vi "Monitor.vi"(8 "Error Out 2":errorcluster, 9 "notifier out 2":refnum<notifier>, 10 "filename":string="Test") -> (0 "Error Out":errorcluster, 2 "output file path":path)   [LabVIEW 2016]
uses:
  <userlib>/Levylab/Lockin-Multichannel/Instrument.Lockin/Instrument.Lockin.lvclass
  <vilib>/Utility/file.llb/Write Delimited Spreadsheet (string).vi
  <userlib>/Levylab/LV to ITX/Main/LV to DAT 1D.vi
  <userlib>/Levylab/LV to ITX/LVtoITX.lvclass
panel:
  out "latest notification":bool
  in  "Lockin IP Address UwU":string="130.49.180.51"
  in  "Tab Control":enum32{"Conductance"}(tab)
  in  "Voltage Pairs (+, -,...)":i32[][](array[numeric])=[[0, 1, 1, 2], [2, 3, 4, 3]]
  in  "Current (I-)":i32
  out "Two Terminal Conductance":cluster{"Y":dbl[], "Y":dbl[]}[](graph) caption="XY Graph"
  out "Four Terminal Resistance":cluster{"Y":dbl[], "Y":dbl[]}[](graph) caption="XY Graph"
  in  "Excitation voltage":dbl=0.1
  in  "Reset":bool
  in  "Diff Voltage?":bool
  out "ALL G2T":dbl[][](graph)
  in  "wait (ms)":u32=60
  out "Humidity":dbl=35.08
  out "Temperature":dbl=27.13
  in  "error in (no error)":errorcluster
  in  "stop":bool
  in  "base path":path=path "C:/Users/ansom/Desktop/Monitor/20180205"
  in  "Comments":string="Test"
  in  "folder name":string="monitor cond"
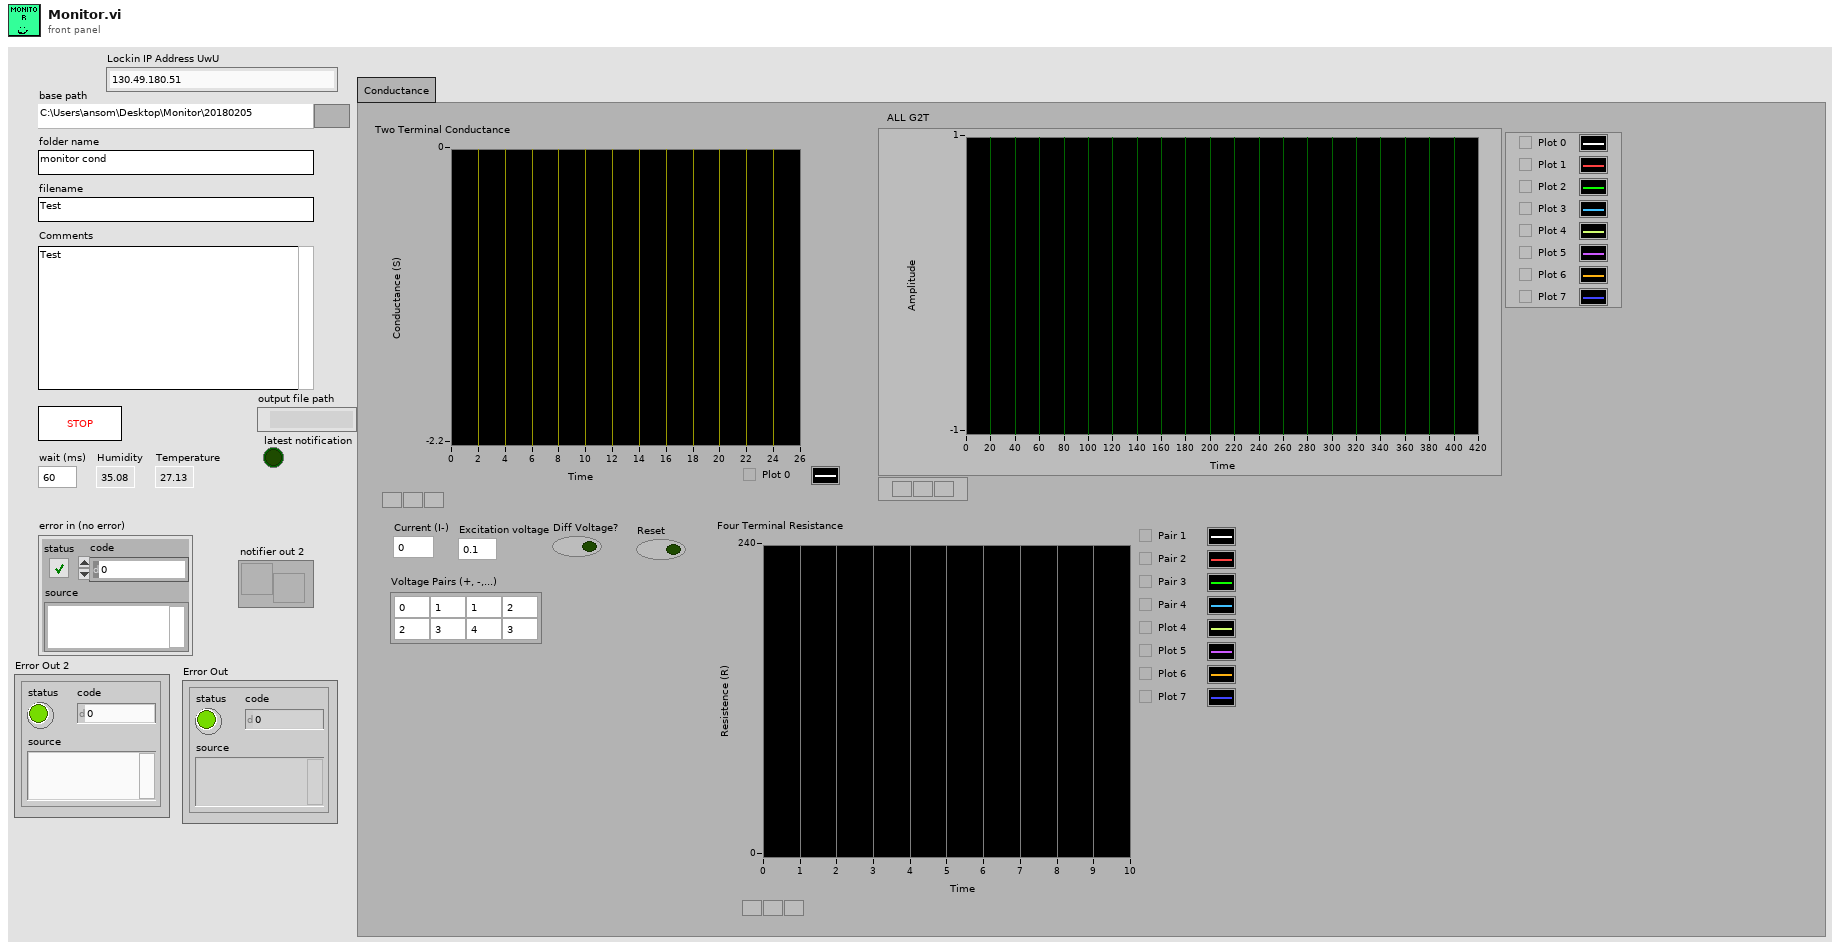
[diagram p1: front panel]
types:
  T1 = enum32{"Bad", "Idle", "Run top level", "Running"}
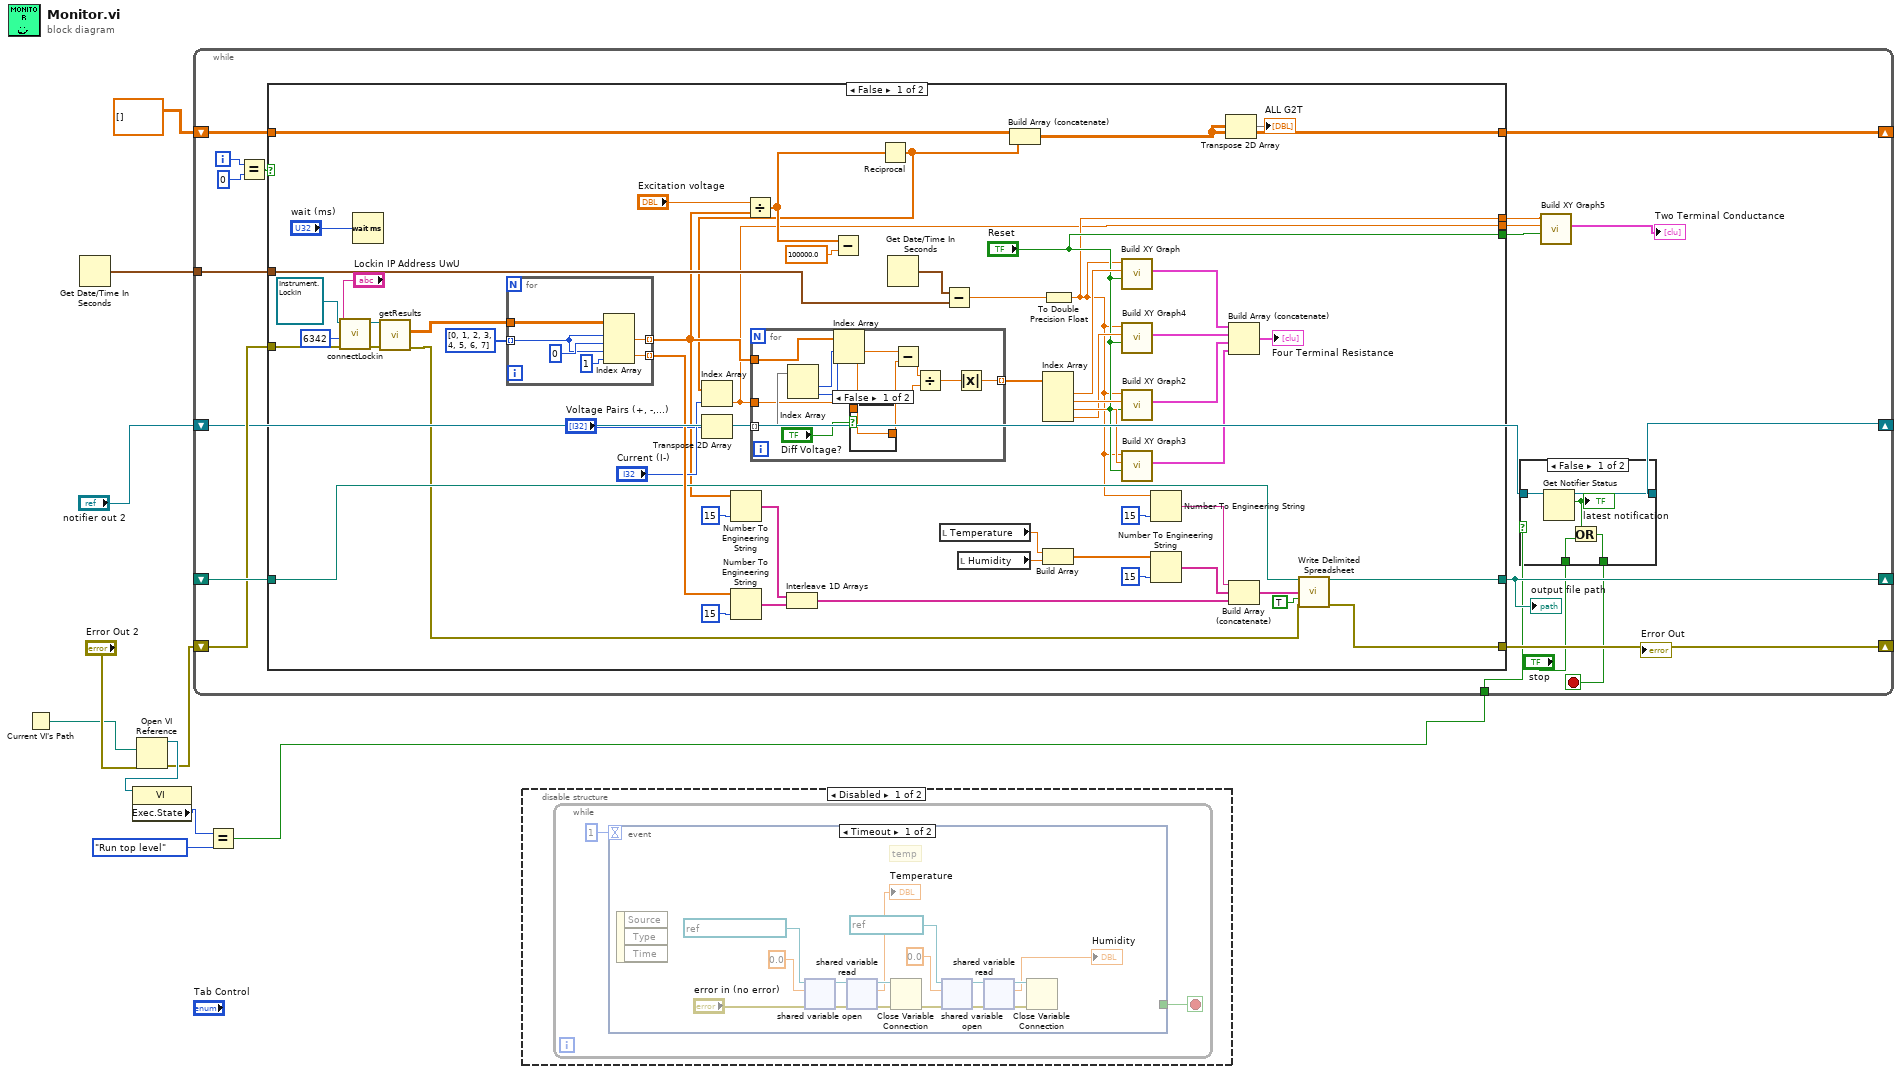
[diagram p0: block diagram]
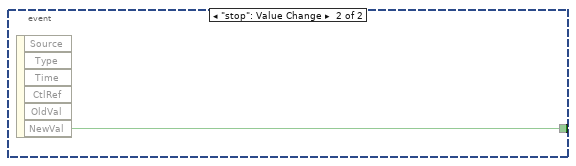
[diagram p2: hidden frame]
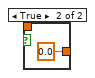
[diagram p5: hidden frame]
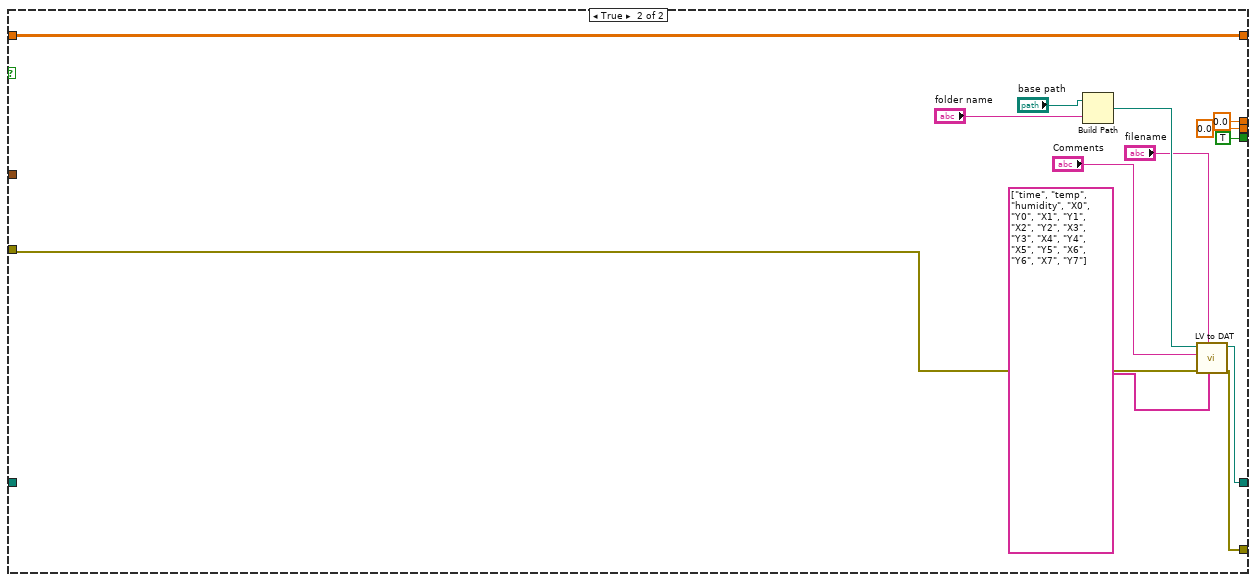
[diagram p6: hidden frame]
diagram:
  n1 = Current VI's Path() -> (path=w1:path)
  n2 = Get Date/Time In Seconds() -> (seconds since 1Jan1904=w11:timestamp)
  n3 = Open VI Reference(vi path=w1, error in (no error)="Error Out 2") -> (vi reference=w7:refnum<vi>, error out=w2:errorcluster)  [unwired: 4 in]
  n4 = property class="VI"(reference=w7) -> ("Exec.State"=w5:T1)  [unwired: 1 in, 2 out]
  n5 = Equal?(x=w5, y=T1."Run top level" ("Execution:State")) -> (x = y?=w3:bool)
  n6 = while {
    shift-right: [w21] -> _
    shift-left: _ -> [w27]
    tunnel: w11 -> [w26]
    shift-right: [w24] -> _
    shift-left: dbl[][] [] ("transposed array") -> [w25]
    shift-right: [w22] -> w9
    shift-left: w2 -> [w23]
    shift-right: [w17] -> _
    shift-left: "notifier out 2" -> [w18]
    tunnel: w3 -> [w19]
    i -> [w30]
    stop <- w16 stop-if-true
    n7 = Equal?(x=w30, y=0) -> (x = y?=w28:bool)
    n8 = case shown="False" w28 {
      tunnel: [w82 w123] -> w21
      tunnel: w27 -> [w85 _]
      tunnel: w26 -> [w58 _]
      tunnel: w25 -> [w50 w118]
      tunnel: [w49 w118] -> w24
      tunnel: w23 -> [w46 w116]
      tunnel: [w45 w117] -> w22
      tunnel: ["Reset" TRUE ("Reset")] -> w15
      tunnel: [w43 0.0] -> w14
      tunnel: [w42 0.0] -> w13
      frame False {
        n9 = call <userlib>:"connectLockin.vi"("error in (no error)"=w46, "Port"=u16 6342, "Address"="Lockin IP Address UwU", "Instrument.Lockin in"=refnum<class "Instrument.Lockin.lvclass"> refnum) -> ("error out"=w39:errorcluster, "Instrument.Lockin out"=w38:refnum<class "Instrument.Lockin.lvclass">)  [unwired: 6 in]
        n10 = Wait (ms)(milliseconds to wait="wait (ms)") -> ()  [unwired: 1 out]
        n11 = call <userlib>:"getResults.vi"("error in (no error)"=w39, "Instrument.Lockin in"=w38) -> ("error out"=w40:errorcluster, "Results"=w41:dbl[][])  [unwired: 6 in, 2 out]
        n12 = for {
          tunnel: w41 -> [w109]
          tunnel: i32[] [0, 1, 2, 3, 4, 5, 6, 7] ("Lockins") -> [w110] mode=indexing
          tunnel: [w107] -> w51 mode=indexing
          tunnel: [w108] -> w86 mode=indexing
          n13 = Index Array(array=w109, index (row) #1=w110, index (col) #1=0 ("disabled index (col)"), index (row) #2=w110, index (col) #2=1 ("disabled index (col)")) -> (element #1=w107:dbl, element #2=w108:dbl)
        }
        n14 = Transpose 2D Array(2D array="Voltage Pairs (+, -,...)") -> (transposed array=w71:i32[][])
        n15 = Number To Engineering String(2:i16 15 ("precision (6)"), 4:w51) -> (0:w89:string[])  [unwired: 2 out]
        n16 = Number To Engineering String(2:i16 15 ("precision (6)"), 4:w86) -> (0:w88:string[])  [unwired: 2 out]
        n17 = Divide(x="Excitation voltage", y=w51) -> (x/y=w55:dbl[])
        n18 = Interleave 1D Arrays(w89, w88) -> (w87:string[])
        n19 = Subtract(x=w55, y=100000.0) -> ()  [unwired: 1 out]
        n20 = Reciprocal(x=w55) -> (1/x=w47:dbl[])
        n21 = Index Array(array=w47, index="Current (I-)") -> (element=w42:dbl)
        n22 = for {
          tunnel: w71 -> [w104] mode=indexing
          tunnel: w51 -> [w103]
          tunnel: w42 -> [w99]
          tunnel: [w96] -> w70 mode=indexing
          n23 = Index Array(array=w104) -> (element #1=w102:i32, element #2=w101:i32)  [unwired: 2 in]
          n24 = Index Array(array=w103, index #1=w102, index #2=w101) -> (element #1=w100:dbl, element #2=w93:dbl)
          n25 = case shown="False" "Diff Voltage?" {
            tunnel: [w105 0.0] -> w94
            tunnel: w93 -> [w105 _]
            frame False {
            }
            frame True {
            }
          }
          n26 = Subtract(x=w100, y=w94) -> (x-y=w98:dbl)
          n27 = Divide(x=w98, y=w99) -> (x/y=w97:dbl)
          n28 = Absolute Value(x=w97) -> (abs(x)=w96:dbl)
        }
        n29 = Get Date/Time In Seconds() -> (seconds since 1Jan1904=w59:timestamp)
        n30 = local read "Temperature"() -> (w81:dbl)
        n31 = Subtract(x=w59, y=w58) -> (x-y=w57:dbl)
        n32 = local read "Humidity"() -> (w80:dbl)
        n33 = Build Array (concatenate)(w50, w47) -> (w49:dbl[][])
        n34 = Index Array(array=w70) -> (element #1=w69:dbl, element #2=w68:dbl, element #3=w67:dbl, element #4=w66:dbl)  [unwired: 4 in]
        n35 = Build Array(w81, w80) -> (w75:dbl[])
        n36 = To Double Precision Float(number=w57) -> (double precision float=w43:dbl)
        n37 = call "Build XY Graph"("Reset"="Reset", "Y Input"=w69, "X Input"=w43) -> ("XY Graph"=w65:cluster{"Y":dbl[], "Y":dbl[]}[])  [unwired: 2 in, 6 out]
        n38 = call "Build XY Graph4"("Reset"="Reset", "Y Input"=w66, "X Input"=w43) -> ("XY Graph"=w64:cluster{"Y":dbl[], "Y":dbl[]}[])  [unwired: 2 in, 6 out]
        n39 = call "Build XY Graph2"("Reset"="Reset", "Y Input"=w68, "X Input"=w43) -> ("XY Graph"=w63:cluster{"Y":dbl[], "Y":dbl[]}[])  [unwired: 2 in, 6 out]
        n40 = call "Build XY Graph3"("Reset"="Reset", "Y Input"=w67, "X Input"=w43) -> ("XY Graph"=w62:cluster{"Y":dbl[], "Y":dbl[]}[])  [unwired: 2 in, 6 out]
        n41 = Number To Engineering String(2:i16 15 ("precision (6)"), 4:w43) -> (0:w77:string)  [unwired: 2 out]
        n42 = Number To Engineering String(2:i16 15 ("precision (6)"), 4:w75) -> (0:w74:string[])  [unwired: 2 out]
        n43 = Transpose 2D Array(2D array=w49) -> (transposed array=→"ALL G2T":dbl[][])
        n44 = Build Array (concatenate)(w65, w64, w63, w62) -> (→"Four Terminal Resistance":cluster{"Y":dbl[], "Y":dbl[]}[])
        n45 = Build Array (concatenate)(w77, w74, w87) -> (w83:string[])
        n46 = call-poly <vilib>:"Write Delimited Spreadsheet.vi"("file path (dialog if empty)"=w85, "1D data"=w83, "append to file? (new file:F)"=TRUE, "error in (no error)"=w40) -> ("new file path (Not A Path if cancelled)"=w82:path, "error out"=w45:errorcluster)  [unwired: 10 in]
      }
      frame True {
        n47 = Build Path(base path="base path", name or relative path="folder name") -> (appended path=w122:path)
        n48 = call-poly <userlib>:"LV to DAT.vi"("wavenames (.Vx, etc)"=string[] ["time", "temp", "humidity", "X0", "Y0", "X1", "Y1", "X2", "Y2", "X3", "Y3", "X4", "Y4", "X5", "Y5", "X6", "Y6", "X7", "Y7"], "filename"="filename", "error in"=w116, "Comments"="Comments", "path"=w122) -> ("error out"=w117:errorcluster, "new file path"=w123:path)  [unwired: 5 in]
      }
    }
    "output file path" <- w21
    n49 = case shown="False" w19 {
      tunnel: "stop" -> [w35 w37]
      tunnel: [w34 w37] -> w16
      tunnel: w18 -> [w33 w36]
      tunnel: [w32 w36] -> w17
      frame False {
        n50 = Get Notifier Status(notifier=w33) -> (notifier out=w32:refnum<notifier>, current notification=w31:bool)  [unwired: 1 in, 3 out]
        "latest notification" <- w31
        n51 = Or(x=w31, y=w35) -> (x .or. y?=w34:bool)
      }
      frame True {
      }
    }
    n52 = call "Build XY Graph5"("Reset"=w15, "Y Input"=w13, "X Input"=w14) -> ("XY Graph"=→"Two Terminal Conductance":cluster{"Y":dbl[], "Y":dbl[]}[])  [unwired: 2 in, 6 out]
  }
  "Error Out" <- w9
  n53 = disable-structure shown="Disabled" {
    frame Disabled {
      n54 = while {
        stop <- w127 stop-if-true
        n55 = event shown="[0] Timeout" {
          selector: _ -> [_ _]
          dyn-events: _ -> [_ _]
          timeout: 1 -> [_ _]
          tunnel: [_ w144] -> w127
          event Timeout {
            # "temp"
            n56 = event-data() -> ()  [unwired: 1 in, 3 out]
            n57 = shared-variable-open(refnum<k21> "ni.var.psp://housesoftheholy/MFP3D/MFP3D Temperature" ("shared variable refnum in"), "error in (no error)", 0.0 ("Excitation voltage 2")) -> (w143:refnum<k21>, w142:errorcluster)  [unwired: 1 in]
            n58 = shared-variable-read(w143, w142) -> (w137:refnum<k21>, w136:errorcluster, →"Temperature":dbl)  [unwired: 1 out]
            n59 = Close Variable Connection(8:w136, 11:w137) -> (0:w130:errorcluster)
            n60 = shared-variable-open(refnum<k21> "ni.var.psp://housesoftheholy/MFP3D/MFP3D Hum" ("shared variable refnum in"), w130, 0.0 ("Excitation voltage 2")) -> (w140:refnum<k21>, w139:errorcluster)  [unwired: 1 in]
            n61 = shared-variable-read(w140, w139) -> (w135:refnum<k21>, w134:errorcluster, →"Humidity":dbl)  [unwired: 1 out]
            n62 = Close Variable Connection(8:w134, 11:w135) -> ()  [unwired: 1 out]
          }
          event "stop": Value Change {
            n63 = event-data() -> ("NewVal"=w144:bool)  [unwired: 1 in, 5 out]
          }
        }
      }
    }
    frame Enabled {
    }
  }
